vi "Get Worksheet Names.vi"(8 "error in (no error)":errorcluster, 11 "workbook in":refnum<class "workbook.lvclass">) -> (0 "error out":errorcluster, 2 "Worksheet Names":string[](array[string]), 3 "workbook out":refnum<class "workbook.lvclass">)   [LabVIEW 2017, in "Excel_Specific.lvlib" / "workbook.lvclass"]
uses:
  workbook.lvclass
  workbook.lvclass/workbook.ctl
  worksheet/Get Worksheet.Name.vi
  worksheet/worksheet.lvclass
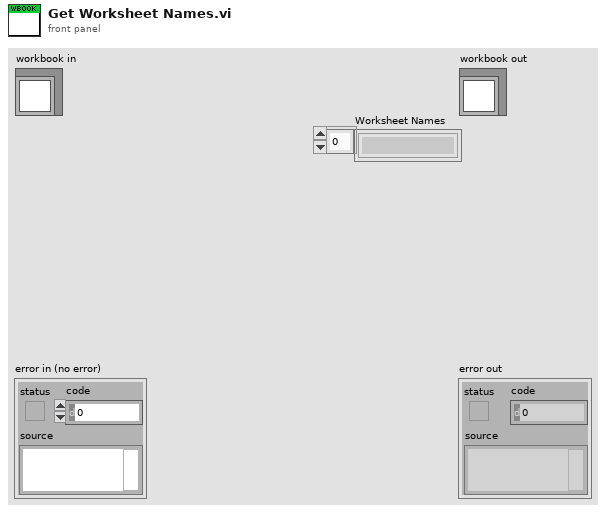
[diagram p1: front panel]
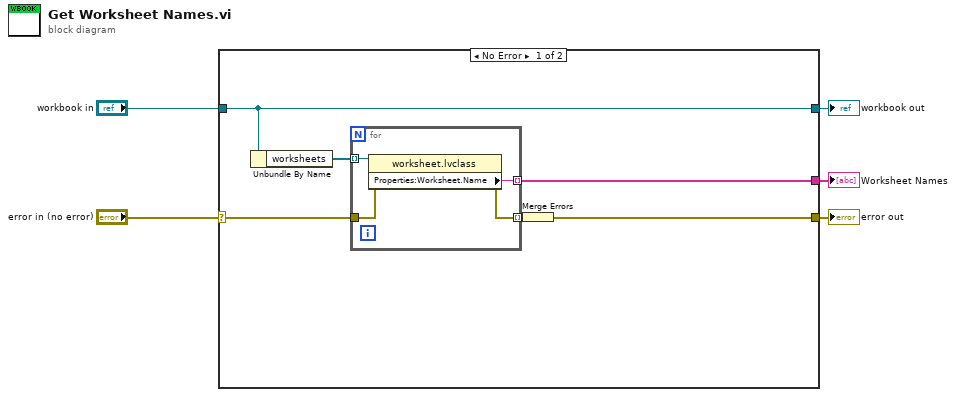
[diagram p0: block diagram]
diagram:
  n1 = case shown="No Error" "error in (no error)" {
    selector: "error in (no error)" -> [w9 w17]
    tunnel: [w6 w17] -> w4
    tunnel: [w10 w16] -> w2
    tunnel: "workbook in" -> [w10 w16]
    tunnel: [w7 _] -> w1
    frame No Error {
      n2 = Unbundle By Name(w10) -> ("worksheets"=w11:refnum<class "worksheet.lvclass">[])
      n3 = for {
        tunnel: w11 -> [w15] mode=indexing
        tunnel: [w14] -> w7 mode=indexing
        tunnel: w9 -> [w13]
        tunnel: [w12] -> w8 mode=indexing
        n4 = property class="worksheet.lvclass"(reference=w15, error in=w13) -> (error out=w12:errorcluster, "Properties:Worksheet.Name"=w14:string)  [unwired: 1 out]
      }
      n5 = Merge Errors(w8) -> (w6:errorcluster)
    }
    frame Error {
    }
  }
  "error out" <- w4
  "workbook out" <- w2
  "Worksheet Names" <- w1
